vi "StimFile (G3)-Initialize.vi"(0 "File":T1, 7 "Npts":i32=-1, 11 "error in (no error)":errorcluster, 12 "Root seed":i32=-1) -> (4 "File out":T1, 15 "error out":errorcluster)   [LabVIEW 2020]
uses:
  Waveform VIs/File VIs/StimFile-Params.ctl
  Utility VIs/Math VIs/LinSpace (x0-dx-npts).vi
  <vilib>/Analysis/1siggen.llb/Riffle Array (I32).vi
  <vilib>/Analysis/NI_AALBase.lvlib
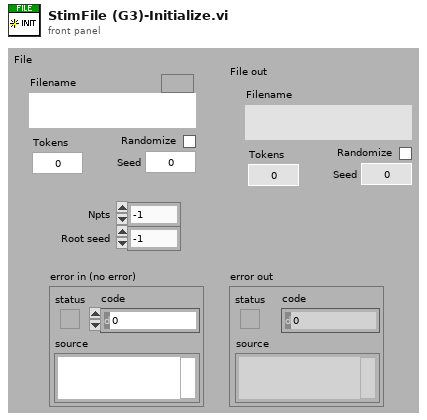
[diagram p1: front panel]
types:
  T1 = typedef "StimFile-Params.ctl" = cluster{"Filename":path, "Signal":dbl[], "Channel":i32, "stream":bool, "offset":i32, "nreps":i32, "loops":i32, "Randomize":bool, "order":i32[], "Seed":i32, "Tokens":i32}
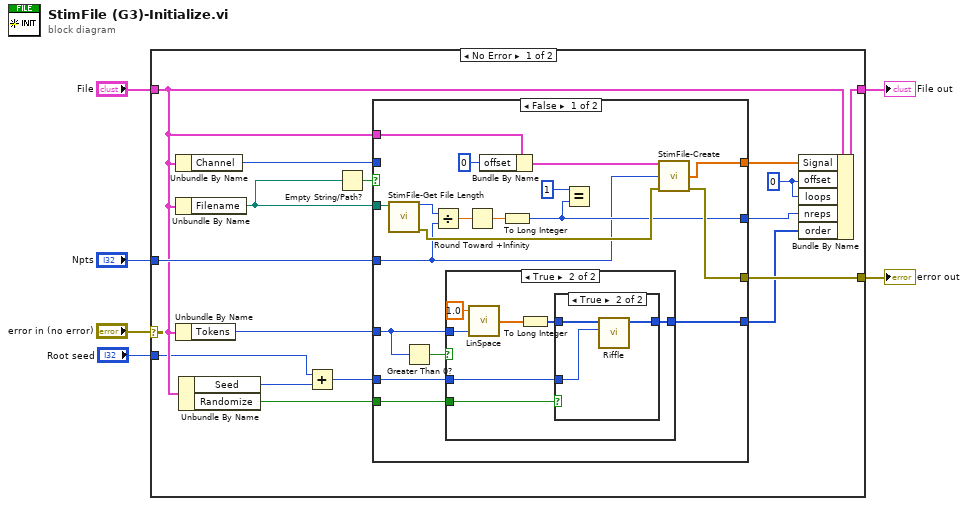
[diagram p0: block diagram]
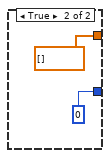
[diagram p4: hidden frame]
diagram:
  n1 = case shown="No Error" "error in (no error)" {
    selector: "error in (no error)" -> [_ w54]
    tunnel: "File" -> [w12 _]
    tunnel: "Npts" -> [w20 _]
    tunnel: [w22 w54] -> w3
    tunnel: [w21 _] -> w2
    tunnel: "Root seed" -> [w7 _]
    frame No Error {
      w14 = 0 ("offset")
      n2 = Unbundle By Name(w12) -> ("Channel"=w16:i32)
      n3 = Unbundle By Name(w12) -> ("Filename"=w17:path)
      n4 = Unbundle By Name(w12) -> ("Tokens"=w13:i32)
      n5 = Unbundle By Name(w12) -> ("Seed"=w9:i32, "Randomize"=w11:bool)
      n6 = Add(x=w7, y=w9) -> (x+y=w8:i32)
      n7 = Empty String/Path?(string/path=w17) -> (empty?=w18:bool)
      n8 = case shown="False" w18 {
        tunnel: w17 -> [w40 _]
        tunnel: [w30 _] -> w22
        tunnel: w20 -> [w28 _]
        tunnel: [w32 dbl[] [] ("Y")] -> w19
        tunnel: w16 -> [_ _]
        tunnel: [w29 0] -> w15
        tunnel: w12 -> [w35 _]
        tunnel: w13 -> [w25 _]
        tunnel: w11 -> [w26 _]
        tunnel: [w24 _] -> w10
        tunnel: w8 -> [w23 _]
        frame False {
          n9 = call "StimFile-Get File Length.vi"("Filename"=w40) -> ("total number of samples/ch"=w39:u32, "error out"=w31:errorcluster)  [unwired: 13 in]
          n10 = Greater Than 0?(x=w25) -> (x > 0?=w27:bool)
          n11 = Divide(x=w39, y=w28) -> (x/y=w38:dbl)
          n12 = case shown="True" w27 {
            tunnel: w26 -> [_ w45]
            tunnel: w25 -> [_ w47]
            tunnel: [_ w44] -> w24
            tunnel: w23 -> [_ w41]
            frame False {
            }
            frame True {
              n13 = call-poly "LinSpace.vi"("npts"=w47, "x0"=1.0) -> ("Array"=w46:dbl[])  [unwired: 2 in, 1 out]
              n14 = To Long Integer(number=w46) -> (32bit integer=w43:i32[])
              n15 = case shown="True" w45 {
                tunnel: [w48 w50] -> w44
                tunnel: w43 -> [w48 w51]
                tunnel: w41 -> [_ w49]
                frame False {
                }
                frame True {
                  n16 = call-poly <vilib>:"Riffle.vi"("seed"=w49, "X"=w51) -> ("Riffled {X}"=w50:i32[])  [unwired: 7 in, 2 out]
                }
              }
            }
          }
          n17 = Round Toward +Infinity(x=w38) -> (ceil(x): smallest int >= x=w37:dbl)
          n18 = Bundle By Name(cluster=w35, "offset"=0) -> (w33:T1)
          n19 = To Long Integer(number=w37) -> (32bit integer=w29:i32)
          n20 = Equal?(x=1, y=w29) -> ()  [unwired: 1 out]
          n21 = call "StimFile-Create.vi"("File"=w33, "Npts"=w28, "error in (no error)"=w31) -> ("Y"=w32:dbl[], "error out"=w30:errorcluster)  [unwired: 10 in, 1 out]
        }
        frame True {
        }
      }
      n22 = Bundle By Name(cluster=w12, "Signal"=w19, "offset"=w14, "loops"=w14, "nreps"=w15, "order"=w10) -> (w21:T1)
    }
    frame Error {
    }
  }
  "error out" <- w3
  "File out" <- w2
